vi "eGateHSP_ReadBuffer.vi"(6 "Fehler (Eingang, kein Fehler)":errorcluster, 9 "e.gate Configuration":T1 {"StartTime" format="%#.10f"; "dActTimeToSecondFactor" format="%#.10f"; "StartTimeToDayFactor" format="%#_10f"}) -> (0 "Fehler (Ausgang)":errorcluster, 1 "number of Frames":i32, 2 "Array":dbl[][](array[numeric]), 3 "e.gate Configuration 2":T1 {"StartTime" format="%#.10f"; "dActTimeToSecondFactor" format="%#.10f"; "StartTimeToDayFactor" format="%#_10f"})   [LabVIEW 2016]
uses:
  e.gate Configuration.ctl
  e.gate Channel Data.ctl
  e.gate Data Type.ctl
  e.gate Protocol Type.ctl
  e.gate Module  Data.ctl
  e.gateHSP_DLLhandle.ctl
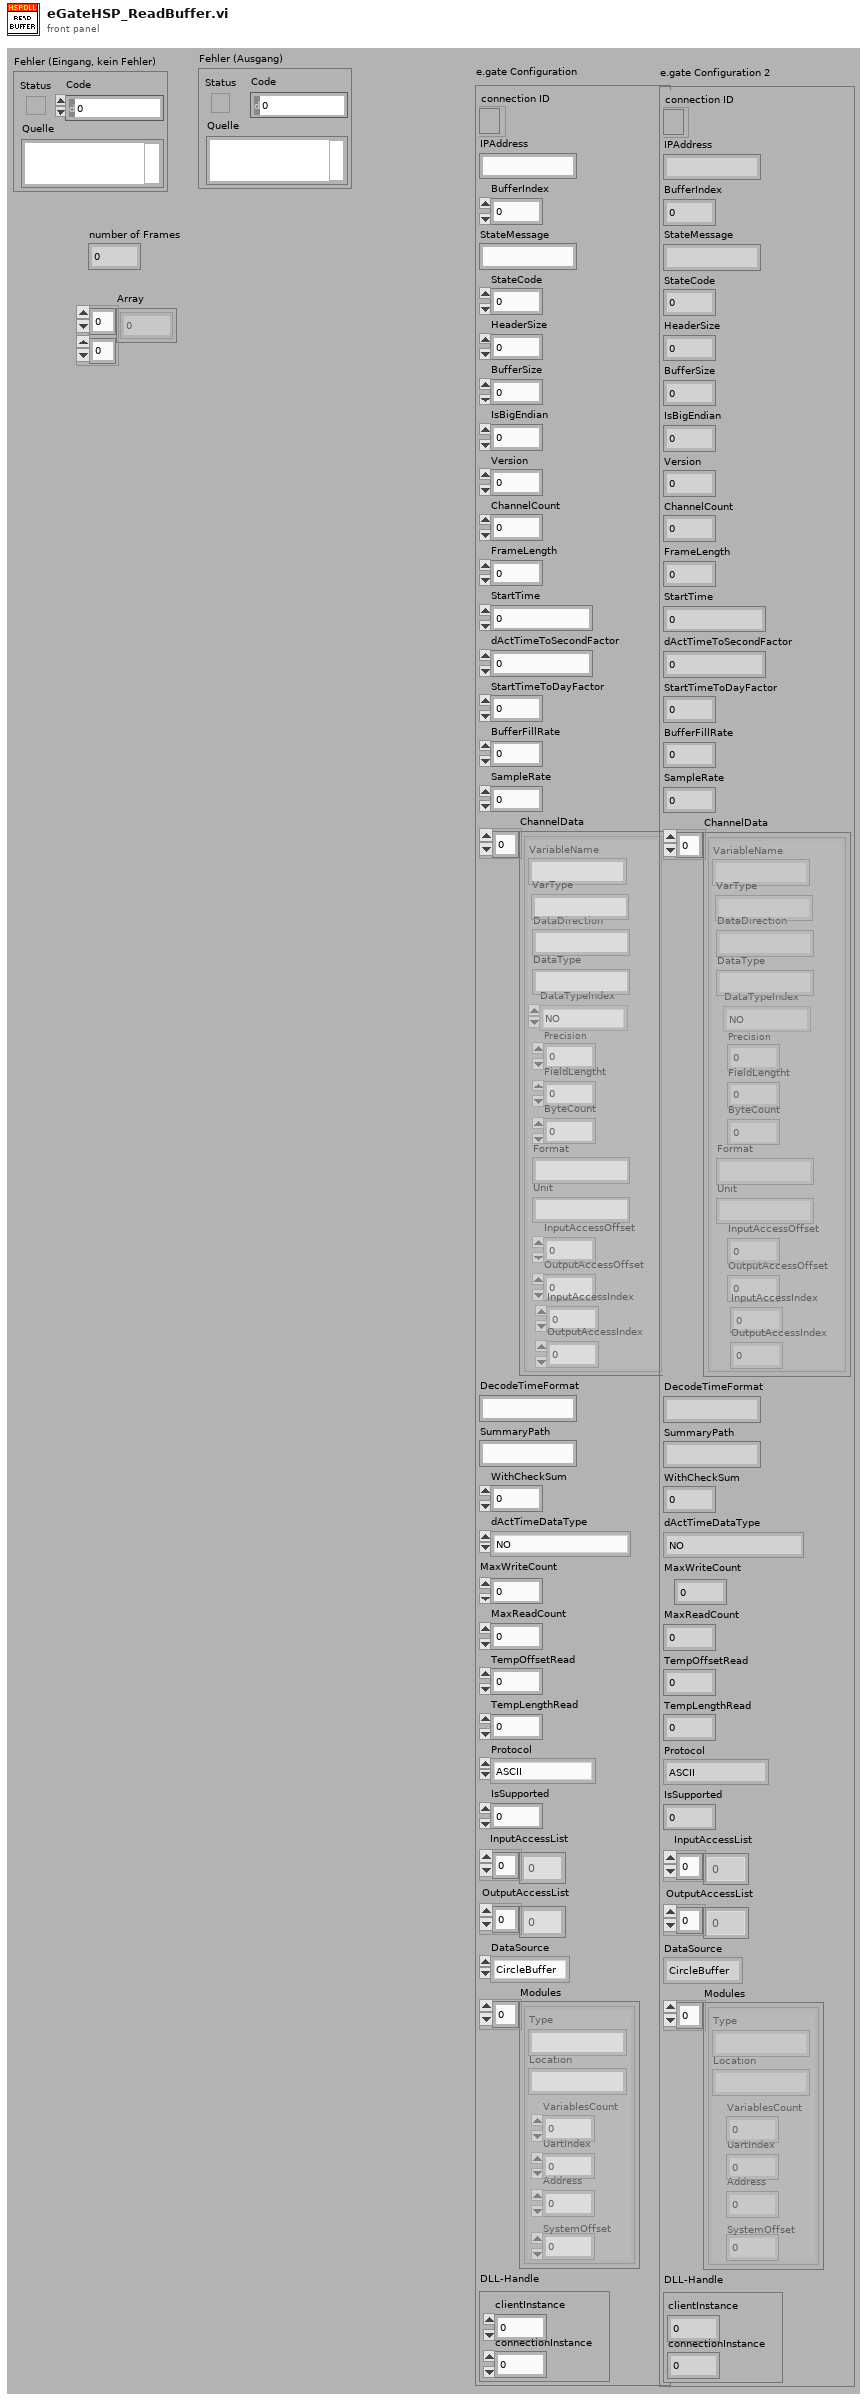
[diagram p1: front panel]
types:
  T1 = typedef "e.gate Configuration.ctl" = cluster{"connection ID":refnum<k5>, "IPAddress":string, "BufferIndex":i32, "StateMessage":string, "StateCode":i8, "HeaderSize":i32, "BufferSize":i32, "IsBigEndian":i32, "Version":i32, "ChannelCount":i32, "FrameLength":i32, "StartTime":dbl, "dActTimeToSecondFactor":dbl, "StartTimeToDayFactor":dbl, "BufferFillRate":dbl, "SampleRate":dbl, "ChannelData":T2[], "DecodeTimeFormat":string, "SummaryPath":string, "WithCheckSum":i32, "dActTimeDataType":T3, "MaxWriteCount":i32, "MaxReadCount":i32, "TempOffsetRead":i32, "TempLengthRead":i32, "Protocol":T4, "IsSupported":i32, "InputAccessList":i32[], "OutputAccessList":i32[], "DataSource":enum16{"CircleBuffer", "test.con Logger", "test.con Archive"}, "Modules":T5[], "DLL-Handle":T6}
  T2 = typedef "e.gate Channel Data.ctl" = cluster{"VariableName":string, "DataDirection":string, "DataType":string, "DataTypeIndex":T3, "Precision":i16, "FieldLengtht":i16, "ByteCount":i32, "Format":string, "Unit":string, "InputAccessOffset":i32, "OutputAccessOffset":i16, "InputAccessIndex":i16, "OutputAccessIndex":i16, "VarType":string}
  T3 = typedef "e.gate Data Type.ctl" = enum16{"NO", "BOOL", "SINT8", "USINT8", "SINT16", "USINT16", "SINT32", "USINT32", "FLOAT", "SET8", "SET16", "SET32", "DOUBLE", "SINT64", "USINT64", "SET64"}
  T4 = typedef "e.gate Protocol Type.ctl" = enum16{"ASCII", "HighspeedPort Online", "HighspeedPort Buffer", "eGateHighspeedPortDLL "}
  T5 = typedef "e.gate Module  Data.ctl" = cluster{"Type":string, "Location":string, "VariablesCount":i16, "UartIndex":i16, "Address":i16, "SystemOffset":i16}
  T6 = typedef "e.gateHSP_DLLhandle.ctl" = cluster{"clientInstance":i32, "connectionInstance":i32}
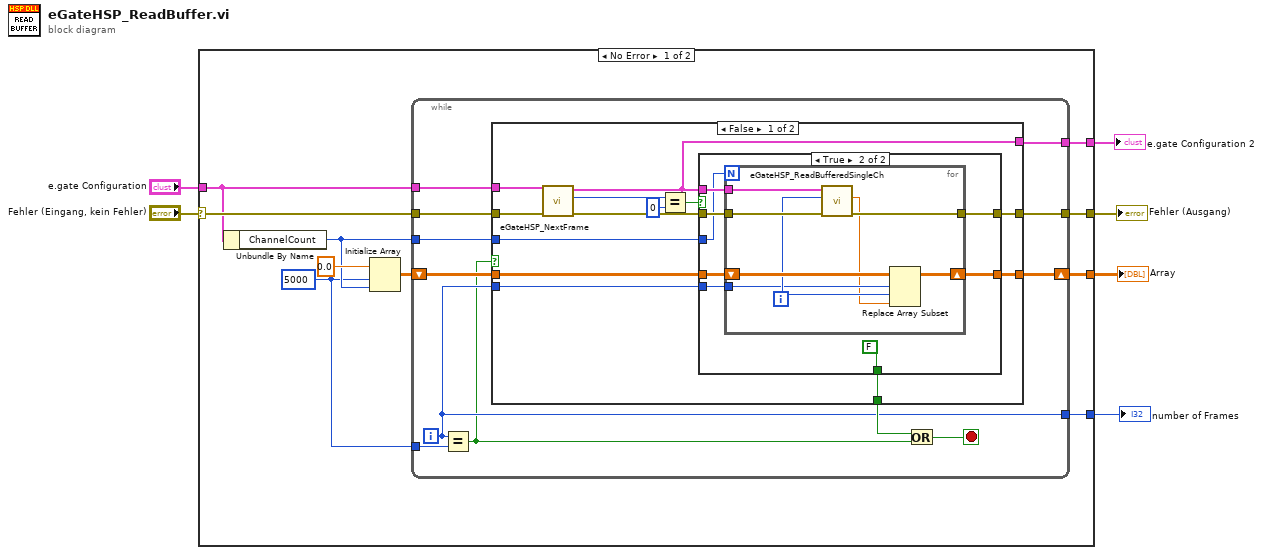
[diagram p0: block diagram]
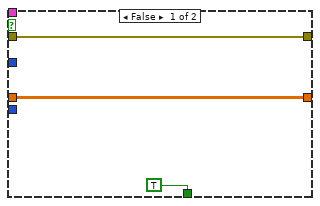
[diagram p2: hidden frame]
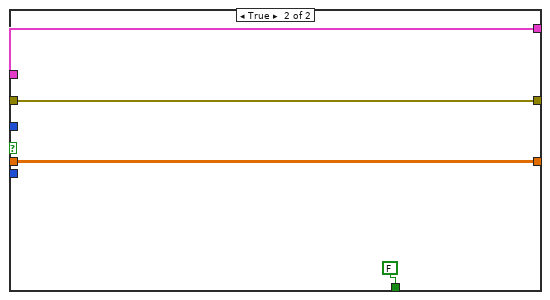
[diagram p3: hidden frame]
diagram:
  n1 = case shown="No Error" "Fehler (Eingang, kein Fehler)" {
    selector: "Fehler (Eingang, kein Fehler)" -> [w16 w65]
    tunnel: "e.gate Configuration" -> [w15 _]
    tunnel: [w14 w65] -> w4
    tunnel: [w8 _] -> w3
    tunnel: [w9 _] -> w2
    tunnel: [w7 _] -> w1
    frame No Error {
      w10 = 5000 ("Dimension")
      n2 = Unbundle By Name(w15) -> ("ChannelCount"=w11:i32)
      n3 = Initialize Array(0.0 ("Element"), w10, w11) -> (w12:dbl[][])
      n4 = while {
        tunnel: w15 -> [w28]
        tunnel: w16 -> [w27]
        tunnel: [w26] -> w14
        tunnel: w10 -> [w22]
        tunnel: [w21] -> w9
        shift-right: [w19] -> w8
        shift-left: w12 -> [w20]
        tunnel: w11 -> [w25]
        tunnel: [w18] -> w7
        i -> [w18]
        stop <- w23 stop-if-true
        n5 = Equal?(x=w18, y=w22) -> (x = y?=w17:bool)
        n6 = case shown="False" w17 {
          tunnel: w28 -> [w41 w64]
          tunnel: w27 -> [w40 w63]
          tunnel: [w36 w63] -> w26
          tunnel: w25 -> [w34 _]
          tunnel: [w33 FALSE] -> w24
          tunnel: [w32 w64] -> w21
          tunnel: w20 -> [w31 w62]
          tunnel: [w30 w62] -> w19
          tunnel: w18 -> [w29 _]
          frame False {
            n7 = call "eGateHSP_NextFrame.vi"("Fehler (Eingang, kein Fehler)"=w40, "e.gate Configuration"=w41) -> ("Fehler (Ausgang)"=w37:errorcluster, "returnvalue"=w39:i32, "e.gate Configuration 2"=w32:T1)  [unwired: 7 in]
            n8 = Equal?(x=w39, y=0) -> (x = y?=w35:bool)
            n9 = case shown="True" w35 {
              tunnel: w32 -> [_ w52]
              tunnel: [TRUE FALSE] -> w33
              tunnel: w37 -> [w43 w50]
              tunnel: [w43 w49] -> w36
              tunnel: w34 -> [_ w48]
              tunnel: w31 -> [w42 w47]
              tunnel: w29 -> [_ w46]
              tunnel: [w42 w45] -> w30
              frame False {
              }
              frame True {
                n10 = for {
                  N: w48 -> [_]
                  tunnel: w52 -> [w60]
                  tunnel: w50 -> [w59]
                  tunnel: [w58] -> w49
                  tunnel: w46 -> [w55]
                  shift-right: [w53] -> w45
                  shift-left: w47 -> [w57]
                  i -> [w56]
                  n11 = call "eGateHSP_ReadBufferedSingleCh.vi"("Fehler (Eingang, kein Fehler)"=w59, "ChannelIndex"=w56, "e.gate Configuration"=w60) -> ("Fehler (Ausgang)"=w58:errorcluster, "value"=w54:dbl)  [unwired: 7 in]
                  n12 = Replace Array Subset(array=w57, new element=w54, index (row)=w55, index (col)=w56) -> (w53:dbl[][])
                }
              }
            }
          }
          frame True {
          }
        }
        n13 = Or(x=w24, y=w17) -> (x .or. y?=w23:bool)
      }
    }
    frame Error {
    }
  }
  "Fehler (Ausgang)" <- w4
  "Array" <- w3
  "e.gate Configuration 2" <- w2
  "number of Frames" <- w1
